vi "uart data_akcelerometr_copy.vi"() -> ()   [LabVIEW 2015]
uses:
  data_typedef.ctl
  <vilib>/Instr/_visa.llb/VISA Configure Serial Port (Instr).vi
panel:
  out "X out":dbl[](array[numeric])
  out "Y out":dbl[](array[numeric])
  out "Z out":dbl[](array[numeric])
  out "Accelero Chart":T1(graph)
  out "Temperature Chart":dbl[](graph)
  out "Accelero Array":dbl[](array[numeric])
  out "Temperature Array":dbl[](array[numeric])
  out "Numeric":i32
  in  "stop":bool
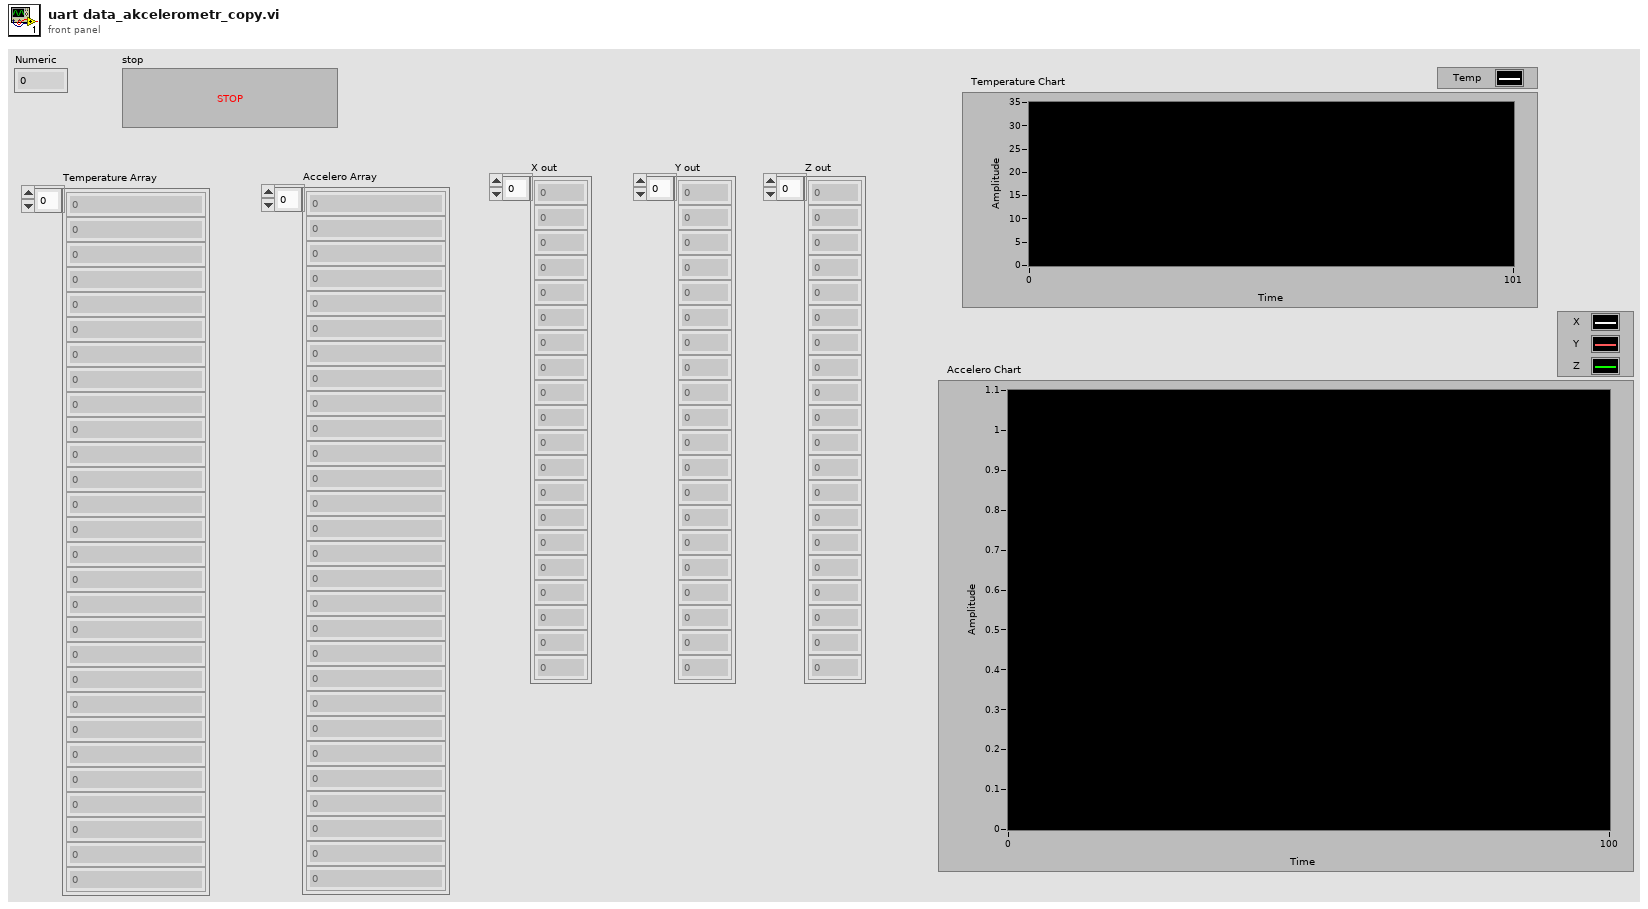
[diagram p1: front panel]
types:
  T1 = cluster{"X element out":dbl, "X element out":dbl, "Z element out":dbl}
  T2 = cluster{"Z element out":dbl, "X element out":dbl, "X element out 2":dbl}[]
  T3 = typedef "data_typedef.ctl" = cluster{"Accelero Array":dbl[], "Z out":dbl[], "Y out":dbl[], "X out":dbl[], "Numeric":i32}
  T4 = typedef "enum_typedef.ctl" = enum16{"Temperature", "X axis", "Y axis", "Z axis"}
  T5 = cluster{"X element out":dbl, "Y element out":dbl, "Z element out":dbl}
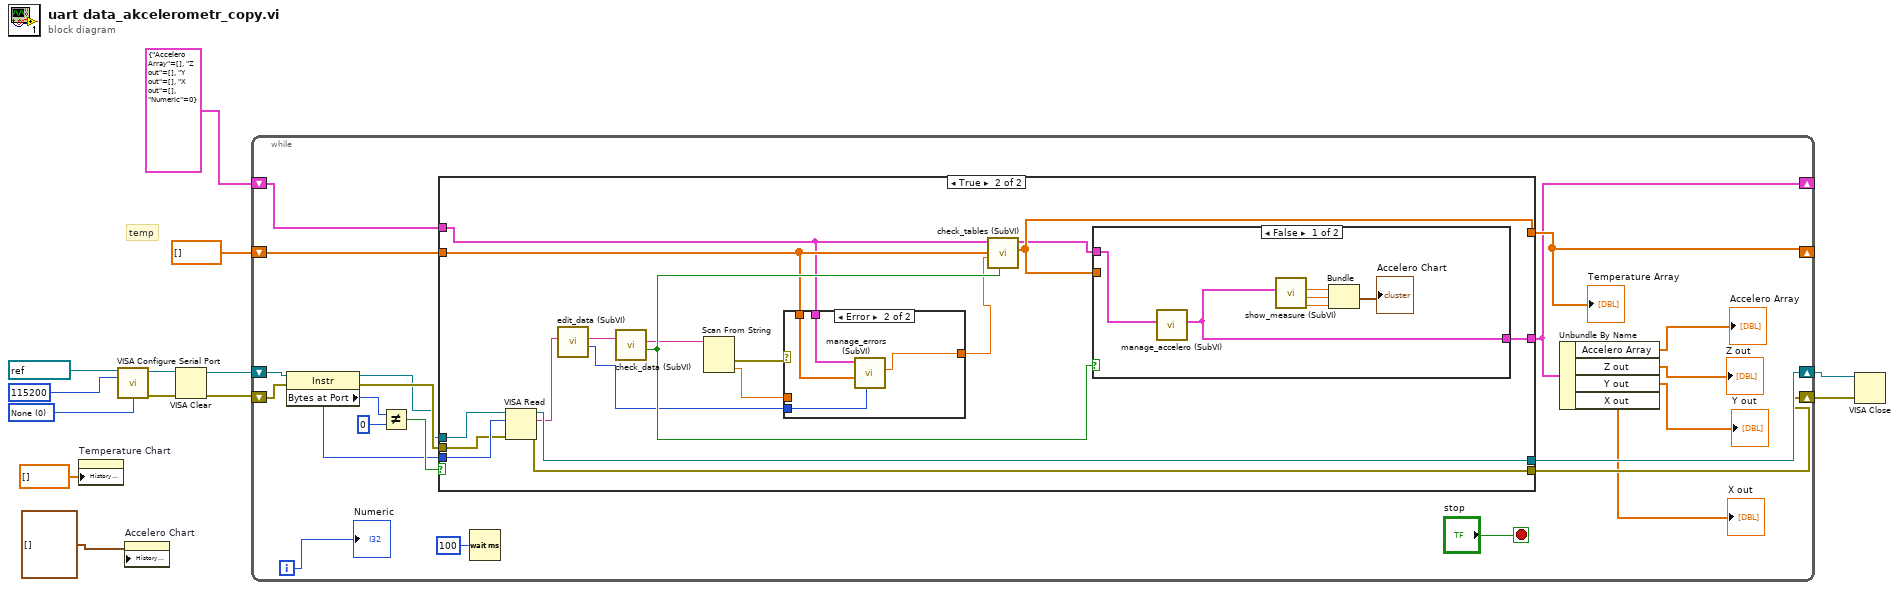
[diagram p0: block diagram]
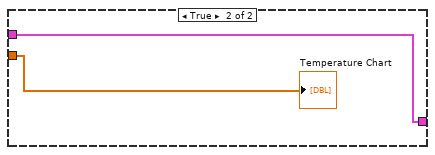
[diagram p4: hidden frame]
diagram:
  w9 = u16 0 items=["None", "XON/XOFF", "RTS/CTS", "XON/XOFF & RTS/CTS", "DTR/DSR", "XON/XOFF & DTR/DSR"] ("flow control (0:none)")
  # "temp"
  n1 = property on="Temperature Chart" class="WFChart (strict)"("History Data"=dbl[] []) -> ()  [unwired: 2 in, 2 out]
  n2 = call-poly "VISA Configure Serial Port"("VISA resource name"=refnum<visa-resource-name> "COM5", "baud rate (9600)"=u32 115200, "flow control (0:none)"=w9) -> ("VISA resource name out"=w5:refnum<visa-resource-name>, "error out"=w4:errorcluster)  [unwired: 11 in]
  n3 = property on="Accelero Chart" class="WFChart (strict)"("History Data"=T2 []) -> ()  [unwired: 2 in, 2 out]
  n4 = VISA Clear(VISA resource name=w5, error in (no error)=w4) -> (VISA resource name out=w6:refnum<visa-resource-name>, error out=w7:errorcluster)
  n5 = while {
    shift-right: [w32] -> w11
    shift-left: w6 -> [w31]
    shift-right: [w28] -> w10
    shift-left: w7 -> [w29]
    shift-right: [w21] -> _
    shift-left: dbl[] [] -> [w24]
    shift-right: [w18] -> _
    shift-left: T3 {"Accelero Array"=[], "Z out"=[], "Y out"=[], "X out"=[], "Numeric"=0} ("Tabs") -> [w19]
    i -> [w20]
    stop <- "stop" stop-if-true
    # "main loop"
    n6 = property class="Instr"(reference=w31, error in=w29) -> (reference out=w27:refnum<visa-resource-name>, error out=w30:errorcluster, "Bytes at Port"=w23:u32)
    n7 = Not Equal?(x=w23, y=u32 0) -> (x != y?=w25:bool)
    n8 = case shown="True" w25 {
      tunnel: [w37 w55] -> w32
      tunnel: w23 -> [_ w54]
      tunnel: w30 -> [w36 w53]
      tunnel: [w36 w52] -> w28
      tunnel: w27 -> [w37 w51]
      tunnel: w24 -> [w35 w39]
      tunnel: [w35 w47] -> w21
      tunnel: w19 -> [w34 w38]
      tunnel: [w34 w46] -> w18
      frame False {
      }
      frame True {
        # "true"
        n9 = VISA Read(VISA resource name=w51, byte count=w54, error in (no error)=w53) -> (VISA resource name out=w55:refnum<visa-resource-name>, read buffer=w50:string, error out=w52:errorcluster)  [unwired: 1 out]
        n10 = call "edit_data (SubVI).vi"("data in"=w50) -> ("Enum"=w40:T4, "data out"=w49:string)  [unwired: 9 in]
        n11 = call "check_data (SubVI).vi"("read buffer"=w49) -> ("buffer out"=w45:string, "bool out"=w48:bool)  [unwired: 8 in]
        n12 = Scan From String(input string=w45) -> (error out=w43:errorcluster, output 1=w42:dbl)  [unwired: 4 in, 2 out]
        n13 = case shown="Error" w43 {
          tunnel: w42 -> [w56 _]
          tunnel: [w56 w57] -> w41
          tunnel: w40 -> [_ w60]
          tunnel: w39 -> [_ w59]
          tunnel: w38 -> [_ w58]
          frame No Error {
          }
          frame Error {
            n14 = call "manage_errors (SubVI).vi"("Enum"=w60, "Temperature Array"=w59, "Data in"=w58) -> ("Out value"=w57:dbl)  [unwired: 8 in]
          }
        }
        n15 = call "check_tables (SubVI).vi"("bool in"=w48, "numeric buffer in"=w41, "temperature array in"=w39, "Data in"=w38) -> ("temperature array out"=w47:dbl[], "Data out"=w44:T3)  [unwired: 6 in]
        n16 = case shown="False" w48 {
          tunnel: w47 -> [_ w68]
          tunnel: w44 -> [w62 w67]
          tunnel: [w61 w67] -> w46
          frame False {
            n17 = call "manage_accelero (SubVI).vi"("Data in"=w62) -> ("Data out"=w61:T3)  [unwired: 9 in]
            n18 = call "show_measure (SubVI).vi"("Data in"=w61) -> ("Z element out"=w65:dbl, "Y element out"=w63:dbl, "X element out"=w66:dbl)  [unwired: 8 in]
            n19 = Bundle("X element out"=w66, "Y element out"=w63, "Z element out"=w65) -> (→"Accelero Chart":T5)  [unwired: 1 in]
          }
          frame True {
            "Temperature Chart" <- w68
          }
        }
      }
    }
    "Temperature Array" <- w21
    n20 = Wait (ms)(milliseconds to wait=u32 100) -> ()  [unwired: 1 out]
    n21 = Unbundle By Name(w18) -> ("Accelero Array"=→"Accelero Array":dbl[], "Z out"=→"Z out":dbl[], "Y out"=→"Y out":dbl[], "X out"=→"X out":dbl[])
    "Numeric" <- w20
  }
  n22 = VISA Close(VISA resource name=w11, error in (no error)=w10) -> ()  [unwired: 1 out]
